vi "initializtion.vi"(0 "Fluidofinterest":string="PROPANE.FLD", 1 "path":string, 6 "Clear Memory":bool) -> (14 "refprop _main_directory":string, 15 "Molecular Weight":dbl, 16 "Critical temperature (K)":dbl, 17 "Critical Pressure (kPa)":dbl, 18 "Component Molar Fractions":dbl[](array[numeric]), 19 "Components":i32)   [LabVIEW 2017]
doc: "Please feel free to contact me if you have any questions .\nMy mail:ken_pop@tom.com yan.ding@jci.com"
uses:
  hrf enum_d.ctl
  Mixture Composition cluster_d.ctl
panel:
  out "memory counter":i32
  in  "path 2":string="D:\\ni files\\refproplv\\cll_refprop_dll_on_lv"
  out "Mixure Cluster out":T1
  out "hmx_pathout":path
  in  "error in (no error)":errorcluster
  in  "ReferenceState(hrf)":T2
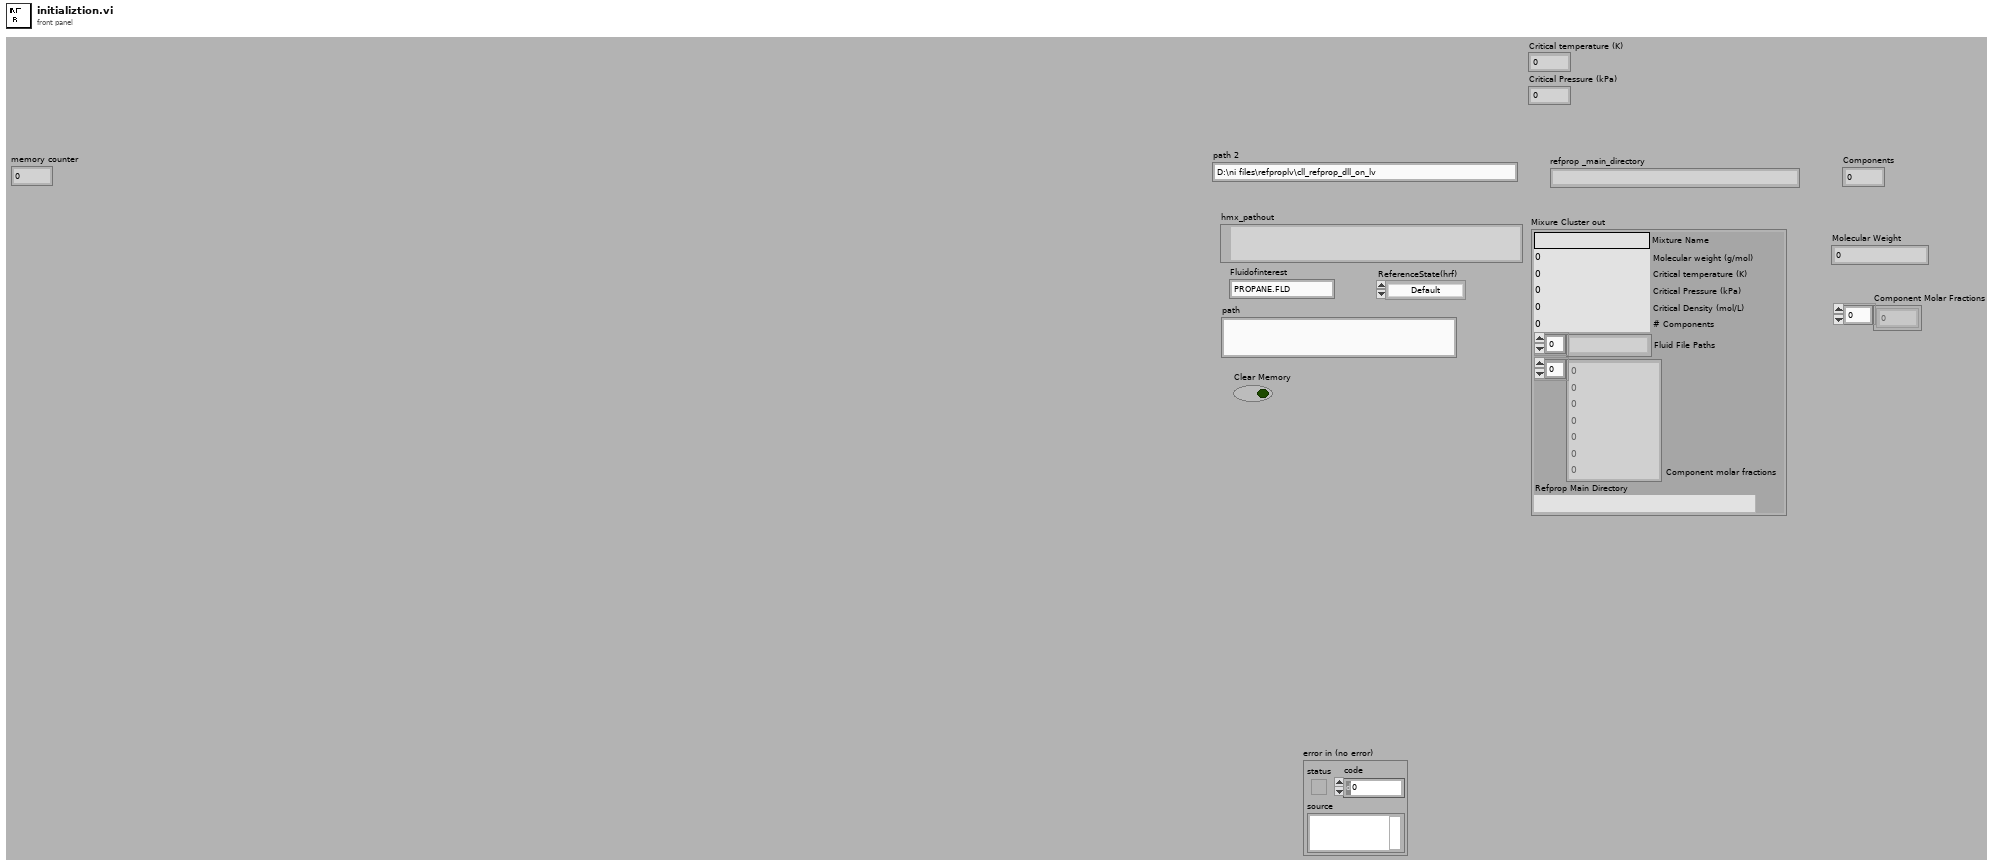
[diagram p1: front panel]
types:
  T1 = typedef "Mixture Composition cluster_d.ctl" = cluster{"Mixture Name":string, "Molecular weight (g/mol)":dbl, "Critical temperature (K)":dbl, "Critical Pressure (kPa)":dbl, "Critical Density (mol/L)":dbl, "# Components":i32, "Fluid File Paths":path[], "Component molar fractions":dbl[], "Refprop Main Directory":path}
  T2 = typedef "hrf enum_d.ctl" = enum16{"Default", "ASHRAE", "IIR"}
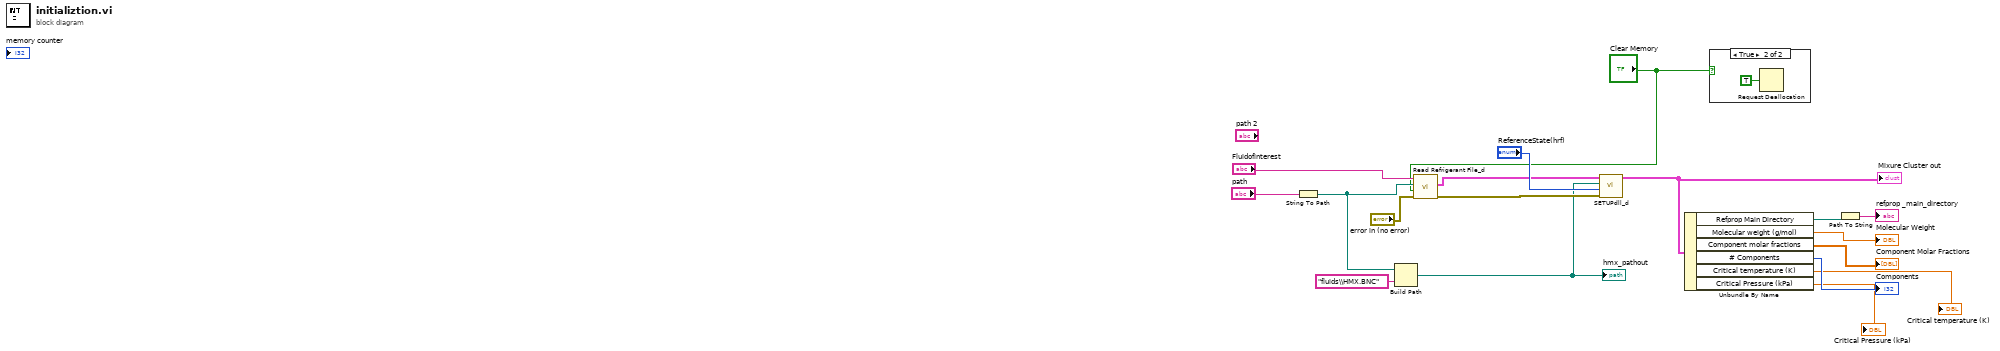
[diagram p0: block diagram]
diagram:
  n1 = String To Path(string="path") -> (path=w13:path)
  n2 = Build Path(base path=w13, name or relative path="fluids\\HMX.BNC" ("名称或相对路径")) -> (appended path=w11:path)
  "hmx_pathout" <- w11
  n3 = call "Read Refrigerant File_d.vi"("error in (no error)"="error in (no error)", "Clear Memory"="Clear Memory", "Refprop Main Directory"=w13, "Refrigerant File"="Fluidofinterest") -> ("error out"=w17:errorcluster, "Mixure Cluster"=w10:T1)  [unwired: 4 in]
  n4 = call "SETUPdll_d.vi"("error in (no error)"=w17, "Reference State (hrf)"="ReferenceState(hrf)", "Path to Mixture file (hfmix)"=w11, "Mixure Cluster in"=w10) -> ("Mixure Cluster out"=w3:T1)  [unwired: 4 in, 1 out]
  "Mixure Cluster out" <- w3
  n5 = Unbundle By Name(w3) -> ("Refprop Main Directory"=w9:path, "Molecular weight (g/mol)"=→"Molecular Weight":dbl, "Component molar fractions"=→"Component Molar Fractions":dbl[], "# Components"=→"Components":i32, "Critical temperature (K)"=→"Critical temperature (K)":dbl, "Critical Pressure (kPa)"=→"Critical Pressure (kPa)":dbl)
  n6 = case shown="True" "Clear Memory" {
    frame False {
    }
    frame True {
      n7 = Request Deallocation(TRUE ("标志")) -> ()
    }
  }
  n8 = Path To String(path=w9) -> (string=→"refprop _main_directory":string)
